vi "Problem 6.vi"(11 "Max Num to Sum Square Diff.":u64=100) -> (3 "Answer":u64)   [LabVIEW 2013, in "Problem 6.lvlib"]
uses:
  Problem 6.lvlib
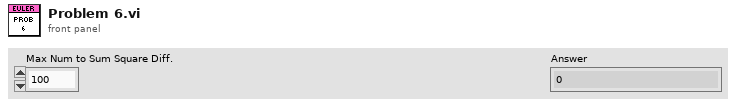
[diagram p1: front panel]
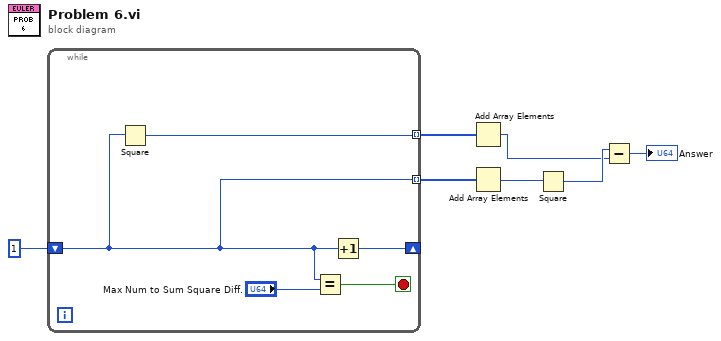
[diagram p0: block diagram]
diagram:
  n1 = while {
    shift-right: [w12] -> _
    shift-left: u64 1 -> [w8]
    tunnel: [w9] -> w6 mode=indexing
    tunnel: [w8] -> w5 mode=indexing
    stop <- w10 stop-if-true
    n2 = Square(x=w8) -> (x^2=w9:u64)
    n3 = Equal?(x=w8, y="Max Num to Sum Square Diff.") -> (x = y?=w10:bool)
    n4 = Increment(x=w8) -> (x+1=w12:u64)
  }
  n5 = Add Array Elements(numeric array=w6) -> (sum=w1:u64)
  n6 = Add Array Elements(numeric array=w5) -> (sum=w4:u64)
  n7 = Square(x=w4) -> (x^2=w2:u64)
  n8 = Subtract(x=w2, y=w1) -> (x-y=→"Answer":u64)
